vi "Write Number of Averages.vi"(8 "error in (no error)":errorcluster, 10 "number of averages":i32=10, 11 "SV Signal in":refnum<class "SV Signal.lvclass">) -> (0 "error out":errorcluster, 3 "SV Signal out":refnum<class "SV Signal.lvclass">)   [LabVIEW 2017, in "SV Signal.lvclass"]
uses:
  <vilib>/addons/_NISVFA/_Generation/Signal Generation/SV Signal/SV Signal.lvclass
  <vilib>/addons/_NISVFA/_Generation/Signal Generation/SV Signal/SV Signal.lvclass/SV Signal.ctl
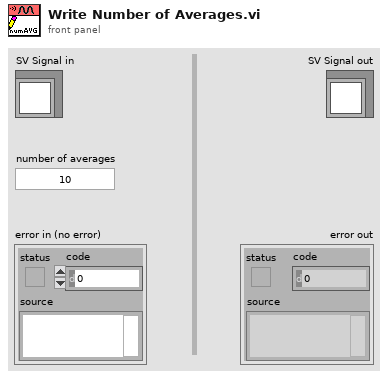
[diagram p1: front panel]
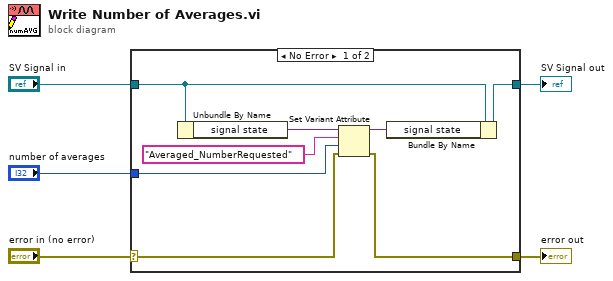
[diagram p0: block diagram]
diagram:
  n1 = case shown="No Error" "error in (no error)" {
    selector: "error in (no error)" -> [w7 w14]
    tunnel: [w6 w14] -> w4
    tunnel: [w13 w15] -> w2
    tunnel: "SV Signal in" -> [w12 w15]
    tunnel: "number of averages" -> [w9 _]
    frame No Error {
      n2 = Unbundle By Name(w12) -> ("signal state"=w11:variant)
      n3 = Set Variant Attribute(Variant=w11, name="Averaged_NumberRequested", value=w9, error in=w7) -> (Variant out=w10:variant, error out=w6:errorcluster)  [unwired: 1 out]
      n4 = Bundle By Name(cluster=w12, "signal state"=w10) -> (w13:refnum<class "SV Signal.lvclass">)
    }
    frame Error {
    }
  }
  "error out" <- w4
  "SV Signal out" <- w2
